vi "Create-Destroy.vi"(8 "Error In":errorcluster) -> (0 "Error Out":errorcluster)   [LabVIEW 2017, in "Tests.lvlib" / "Session.lvlib"]
uses:
  Session.lvlib
  src/LabSSH2/LabSSH2.lvlib
  src/LabSSH2/Public/SSH/Session.lvclass
  <vilib>/addons/_JKI Toolkits/Caraya/classes/Test/Test.lvclass
  <vilib>/addons/_JKI Toolkits/Caraya/classes/Assert/Assert.lvclass
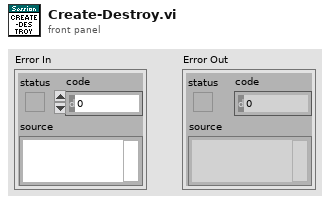
[diagram p1: front panel]
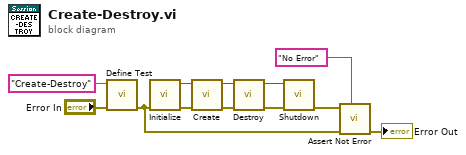
[diagram p0: block diagram]
diagram:
  n1 = call <vilib>:"Define Test.vi"("error in (no error)"="Error In", "Label (VI Title)"="Create-Destroy") -> ("error out"=w5:errorcluster)  [unwired: 9 in]
  n2 = call "Initialize.vi"("Error In"=w5) -> ("Error Out"=w11:errorcluster, "labssh2 Shared Library Out"=w1:path)  [unwired: 9 in]
  n3 = call "Create.vi"("Error In"=w11, "labssh2 Shared Library"=w1) -> ("Error Out"=w9:errorcluster, "Sesssion"=w10:refnum<class "Session.lvclass">)  [unwired: 8 in]
  n4 = call "Destroy.vi"("Error In"=w9, "Session"=w10) -> ("Error Out"=w7:errorcluster, "labssh2 Shared Library"=w8:path)  [unwired: 8 in]
  n5 = call "Shutdown.vi"("Error In"=w7, "labssh2 Shared Library"=w8) -> ("Error Out"=w6:errorcluster)  [unwired: 9 in]
  n6 = call <vilib>:"Assert Not Error.vi"("Label"="No Error", "error in (no error)"=w5, "Not Error?"=w6) -> ("error out"=→"Error Out":errorcluster)  [unwired: 8 in]
